vi "AddParamChannels.vi"(7 "Label Name":string, 8 "error in":errorcluster, 9 "HardwareChannel":i32, 10 "Label Parameters":T2, 11 "Node Ref In":T1=18446744073709551615 format="%.0x") -> (0 "error out":errorcluster, 3 "Node Ref Out":T1=18446744073709551615 format="%.0x")   [LabVIEW 2016, in "Ballard Arinc-429 System Explorer.lvlib"]
uses:
  Ballard Arinc-429 System Explorer.lvlib
  <vilib>/NI Veristand/Custom Device API/Custom Device Item Ref.ctl
  Parse Parameters File/XML_Label.ctl
  Parse Parameters File/XML_Parameter.ctl
  Shared/Controls and Global/Global.vi
  Shared/Ballard Arinc-429 Shared.lvlib
  <vilib>/NI VeriStand/Custom Device API/Custom Device API.lvlib
  <vilib>/NI Veristand/Custom Device API/Set Item Property (U32).vi
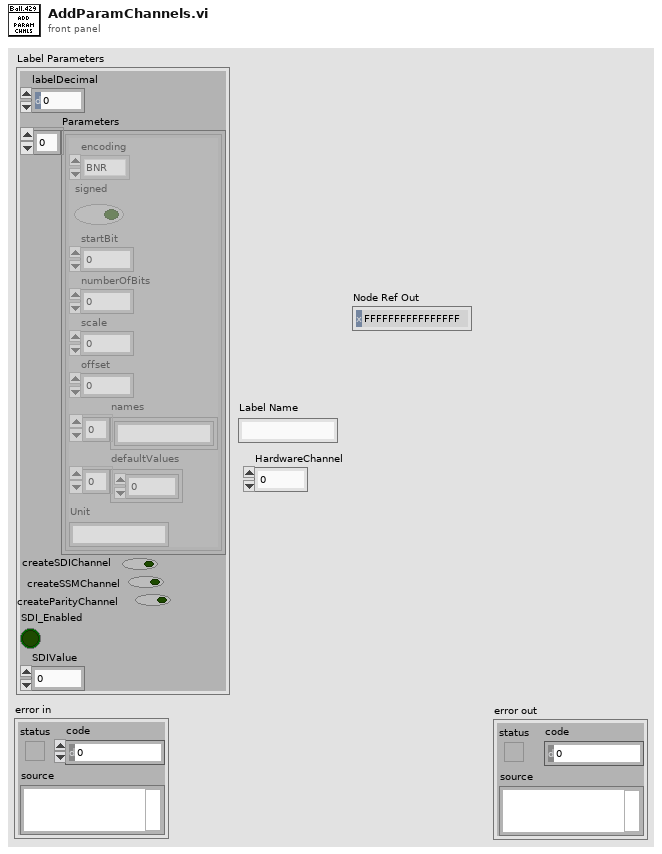
[diagram p1: front panel]
types:
  T1 = typedef "Custom Device API.lvlib/Custom Device Item Ref.ctl" = u64
  T2 = typedef "XML_Label.ctl" = cluster{"labelDecimal":i32, "Parameters":T3[], "createSDIChannel":bool, "createSSMChannel":bool, "createParityChannel":bool, "SDI_Enabled":bool, "SDIValue":u8}
  T3 = typedef "XML_Parameter.ctl" = cluster{"encoding":enum16{"BNR", "BCD", "Discrete"}, "signed":bool, "startBit":i32, "numberOfBits":i32, "scale":dbl, "offset":dbl, "names":string[], "defaultValues":dbl[], "Unit":string}
  T4 = typedef "Custom Device API.lvlib/Custom Device Channel.ctl" = cluster{"Type":T5, "Units":string, "Default Value":dbl, "Faultable":bool, "Scalable":bool}
  T5 = typedef "Custom Device API.lvlib/Custom Device Channel Type.ctl" = enum16{"Input", "Output"}
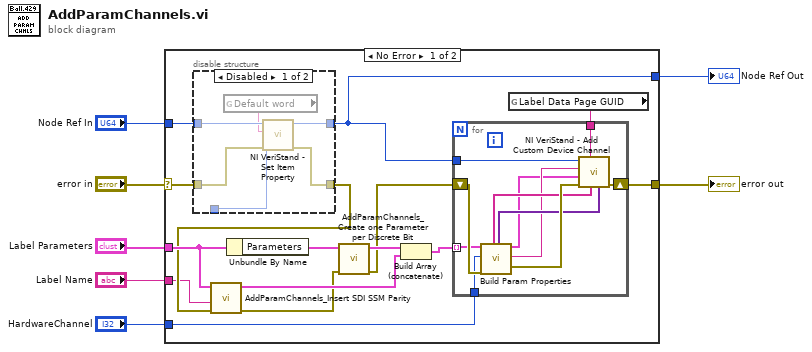
[diagram p0: block diagram]
diagram:
  n1 = case shown="No Error" "error in" {
    selector: "error in" -> [w18 w43]
    tunnel: "Label Parameters" -> [w17 _]
    tunnel: "Node Ref In" -> [w20 w42]
    tunnel: [w21 w43] -> w6
    tunnel: [w19 w42] -> w3
    tunnel: "Label Name" -> [w13 _]
    tunnel: "HardwareChannel" -> [w8 _]
    frame No Error {
      n2 = disable-structure shown="Disabled" {
        disable-tunnel: w20 -> [w28 w29]
        disable-tunnel: [w27 w29] -> w19
        disable-tunnel: w18 -> [w26 w30]
        disable-tunnel: [w25 w30] -> w15
        disable-tunnel: _ -> [w23 _]
        frame Disabled {
          n3 = global read "Global.vi" "Default word"() -> (w24:string)
          n4 = call-poly <vilib>:"NI VeriStand - Set Item Property.vi"("error in (no error)"=w26, "Value"=w23, "Property Name"=w24, "Item Ref in"=w28) -> ("error out"=w25:errorcluster, "Item Ref out"=w27:T1)  [unwired: 5 in, 1 out]
        }
        frame Enabled {
        }
      }
      n5 = call "AddParamChannels_Insert SDI SSM Parity.vi"("error in (no error)"=w15, "Label Name"=w13, "Label Parameters"=w17) -> ("error out"=w10:errorcluster, "Parameters Out"=w16:T3[])  [unwired: 7 in]
      n6 = Unbundle By Name(w17) -> ("Parameters"=w12:T3[])
      n7 = call "AddParamChannels_Create one Parameter per Discrete Bit.vi"("error in (no error)"=w10, "Parameters In"=w12) -> ("error out"=w9:errorcluster, "Parameters Out"=w11:T3[])  [unwired: 8 in]
      n8 = Build Array (concatenate)(w11, w16) -> (w14:T3[])
      n9 = global read "Global.vi" "Label Data Page GUID"() -> (w22:string)
      n10 = for {
        shift-right: [w35] -> w21
        shift-left: w9 -> [w39]
        tunnel: w19 -> [w41]
        tunnel: w22 -> [w40]
        tunnel: w14 -> [w33] mode=indexing
        tunnel: w8 -> [w31]
        n11 = call "Build Param Properties.vi"("Parameter"=w33, "HardwareChannel"=w31, "error in (no error)"=w39) -> ("Prop Names"=w37:string[], "Prop Values"=w36:variant[], "Channel"=w32:T4, "name"=w34:string, "error out"=w38:errorcluster)  [unwired: 7 in, 5 out]
        n12 = call <vilib>:"NI VeriStand - Add Custom Device Channel.vi"("Property Values"=w36, "Property names"=w37, "GUID (Default Channel)"=w40, "error in (no error)"=w38, "Channel"=w32, "Channel Name"=w34, "Parent Ref in"=w41) -> ("error out"=w35:errorcluster)  [unwired: 1 in, 3 out]
      }
    }
    frame Error {
    }
  }
  "error out" <- w6
  "Node Ref Out" <- w3
